vi "DAC.vi"(8 "error in (no error)":errorcluster, 9 "DAC":u8(knob) scale=0.0..255.0, 10 "Pin":u8=25 min=25 max=26, 11 "VISA resource name":refnum<visa-resource-name>) -> (0 "error out":errorcluster, 2 "Voltaje":dbl, 3 "VISA resource name out":refnum<visa-resource-name>)   [LabVIEW 2025]
doc: "Este VI permite usar el DAC de 8 bits que tienen las ESP32, este solo se limita a algunos pines para garantizar su uso \nSe debe ingresar el valor del DAC deseado NO el voltaje \nEl DAC es capaz de suministrar de 0 a 3.3V"
panel:
  out "read buffer":string
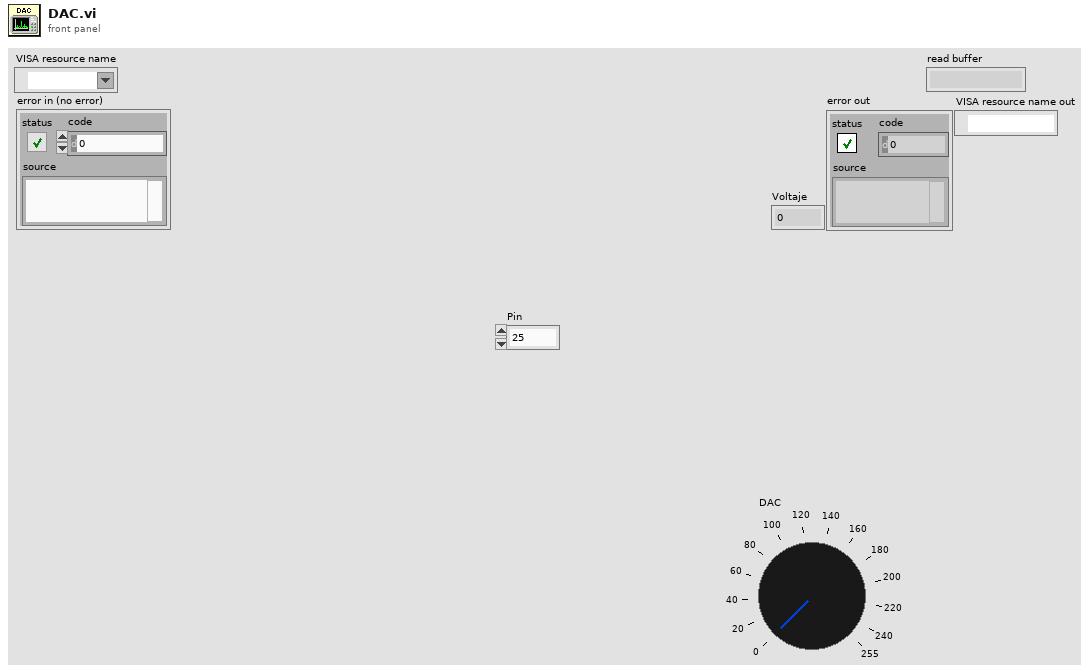
[diagram p1: front panel]
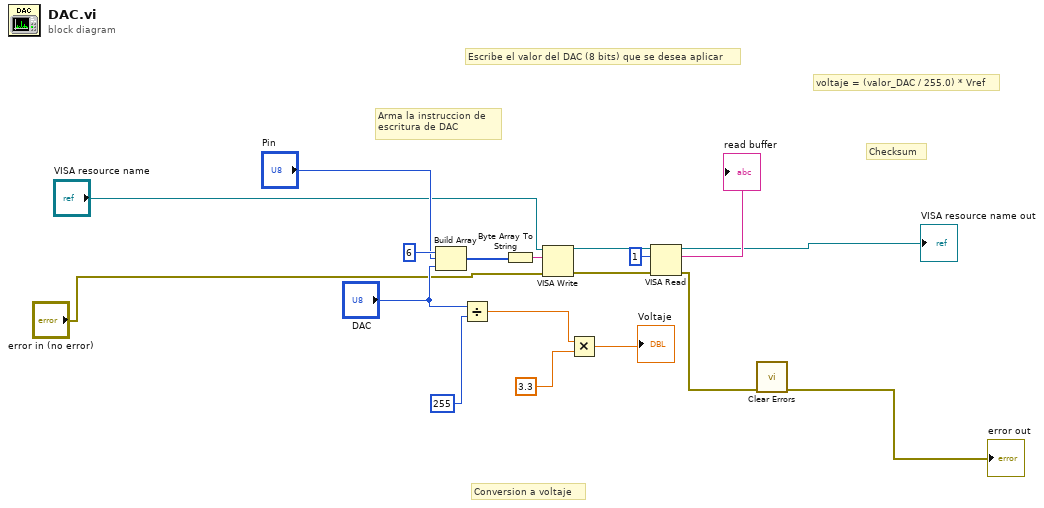
[diagram p0: block diagram]
diagram:
  # "Checksum"
  # "Conversion a voltaje"
  # "Escribe el valor del DAC (8 bits) que se desea aplicar"
  # "Arma la instruccion de \nescritura de DAC"
  # "voltaje = (valor_DAC / 255.0) * Vref"
  n1 = Build Array(u8 6, "Pin", "DAC") -> (w15:u8[])
  n2 = Divide(x="DAC", y=u8 255) -> (x/y=w6:dbl)
  n3 = Byte Array To String(unsigned byte array=w15) -> (string=w18:string)
  n4 = VISA Write(VISA resource name="VISA resource name", write buffer=w18, error in (no error)="error in (no error)") -> (VISA resource name out=w13:refnum<visa-resource-name>, error out=w12:errorcluster)  [unwired: 1 out]
  n5 = Multiply(x=w6, y=3.3) -> (x*y=→"Voltaje":dbl)
  n6 = VISA Read(VISA resource name=w13, byte count=u32 1, error in (no error)=w12) -> (VISA resource name out=→"VISA resource name out":refnum<visa-resource-name>, read buffer=→"read buffer":string, error out=w14:errorcluster)  [unwired: 1 out]
  n7 = call <vilib>:"Clear Errors.vi"("error in (no error)"=w14) -> ("error out"=→"error out":errorcluster)  [unwired: 5 in, 1 out]
